vi "sendValue.vi"(8 "error in (no error)":errorcluster, 10 "data":variant, 11 "errorCode in":refnum<class "errorCode.lvclass">) -> (0 "error out":errorcluster, 2 "function return":i32, 3 "errorCode out":refnum<class "errorCode.lvclass">)   [LabVIEW 2016, in "SALLV_AtDome_Messaging.lvlib" / "errorCode.lvclass"]
uses:
  errorCode.lvclass
  ts_sallv_AtDome/DataTypes/logevent_errorCode.ctl
  errorCode.lvclass/errorCode.ctl
  ts_sallv_AtDome/SALLV_AtDome.lvlib
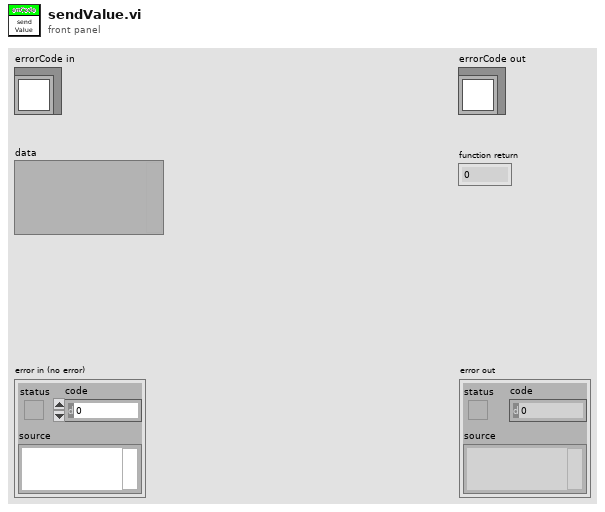
[diagram p1: front panel]
types:
  T1 = typedef "SALLV_AtDome.lvlib/logevent_errorCode.ctl" = cluster{"errorCode":i32, "errorReport":string, "traceback":string, "priority":i32}
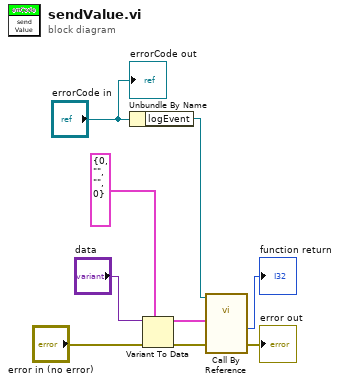
[diagram p0: block diagram]
diagram:
  n1 = Unbundle By Name("errorCode in") -> ("logEvent"=w7:refnum<vi>)
  n2 = Variant To Data(error in="error in (no error)", type=T1 {"errorCode"=0, "errorReport"="", "traceback"="", "priority"=0} ("logevent_errorCode"), Variant="data") -> (data=w1:T1, error out=w5:errorcluster)
  n3 = call-by-ref "?"(reference=w7, "error in (no error)"=w5, "logevent_errorCode_Ctl"=w1) -> ("error out"=→"error out":errorcluster, "function return"=→"function return":i32)  [unwired: 8 in, 3 out]
  "errorCode out" <- "errorCode in"
